vi "GetText.vi"(8 "error in":errorcluster, 11 "TEC editor node in":refnum<class "TEC editor node.lvclass">) -> (0 "error out":errorcluster, 1 "additional text":string, 2 "text":string, 3 "TEC editor node out":refnum<class "TEC editor node.lvclass">, 4 "glyph":string)   [LabVIEW 2013, in "TEC editor node.lvclass"]
uses:
  TEC editor node.lvclass
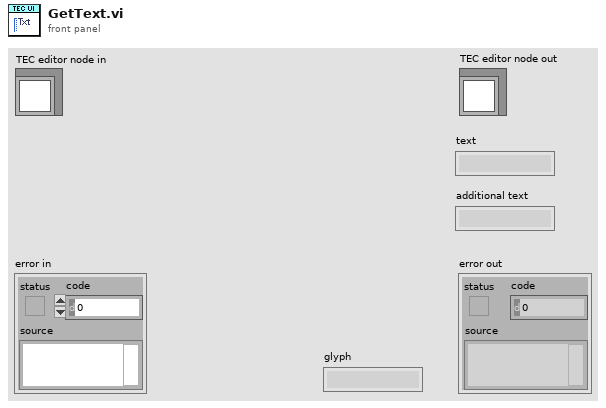
[diagram p1: front panel]
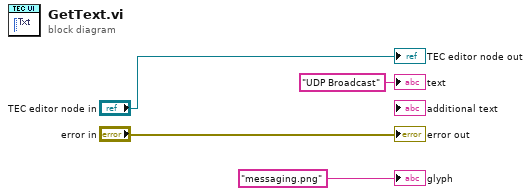
[diagram p0: block diagram]
diagram:
  "error out" <- "error in"
  "TEC editor node out" <- "TEC editor node in"
  "text" <- "UDP Broadcast" ("text")
  "glyph" <- "messaging.png" ("glyph")
